vi "MH_SetHistoOnOff.vi"(8 "error in (no error)":errorcluster, 9 "tacq":i32, 10 "HistoOn/Off":bool, 11 "Multiharp in":refnum<class "Multiharp.lvclass">) -> (0 "error out":errorcluster, 3 "Multiharp out":refnum<class "Multiharp.lvclass">)   [LabVIEW 2023, in "SinglePhoton Library.lvlib" / "Multiharp.lvlib" / "Multiharp.lvclass"]
uses:
  Multiharp.lvclass
  Multiharp.lvclass/Multiharp.ctl
panel:
  in  "event data":T1
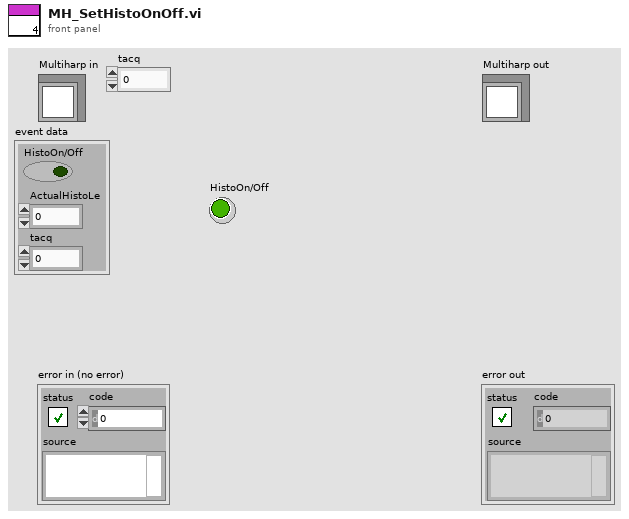
[diagram p1: front panel]
types:
  T1 = cluster{"HistoOn/Off":bool, "ActualHistoLe":i32, "tacq":i32}
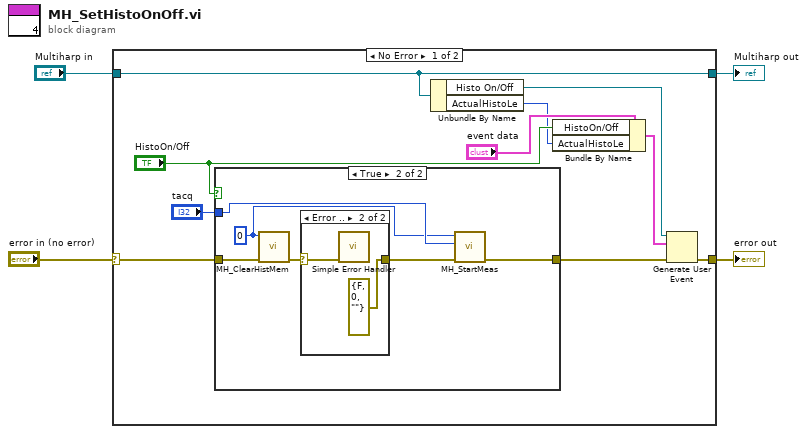
[diagram p0: block diagram]
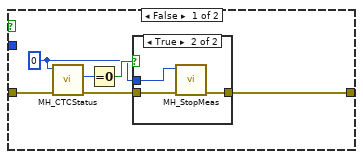
[diagram p2: hidden frame]
diagram:
  n1 = case shown="No Error" "error in (no error)" {
    selector: "error in (no error)" -> [w7 w35]
    tunnel: [w8 w35] -> w3
    tunnel: [w14 w34] -> w1
    tunnel: "Multiharp in" -> [w14 w34]
    frame No Error {
      n2 = case shown="True" "HistoOn/Off" {
        tunnel: [w18 w29] -> w9
        tunnel: w7 -> [w16 w28]
        tunnel: "tacq" -> [_ w30]
        frame False {
          w17 = 0 ("tacq")
          n3 = call "MH_CTCStatus.vi"("error in (no error)"=w16, "devidx"=w17) -> ("error out"=w15:errorcluster, "ctcstatus"=w20:i32)  [unwired: 7 in, 1 out]
          n4 = Equal To 0?(x=w20) -> (x = 0?=w19:bool)
          n5 = case shown="True" w19 {
            tunnel: w17 -> [_ w24]
            tunnel: w15 -> [w21 w23]
            tunnel: [w21 w22] -> w18
            frame False {
            }
            frame True {
              n6 = call "MH_StopMeas.vi"("error in (no error)"=w23, "devidx"=w24) -> ("error out"=w22:errorcluster)  [unwired: 8 in, 1 out]
            }
          }
        }
        frame True {
          w27 = 0 ("devidx")
          n7 = call "MH_ClearHistMem.vi"("error in (no error)"=w28, "devidx"=w27) -> ("error out"=w26:errorcluster)  [unwired: 8 in, 1 out]
          n8 = case shown="Error .." w26 {
            selector: w26 -> [w31 w32]
            tunnel: [w31 errorcluster {"status"=FALSE, "code"=0, "source"=""} ("error IO")] -> w25
            frame No Error {
            }
            frame Error {
              n9 = call <vilib>:"Simple Error Handler.vi"("error in (no error)"=w32) -> ()  [unwired: 4 in, 5 out]
            }
          }
          n10 = call "MH_StartMeas.vi"("error in (no error)"=w25, "tacq"=w30, "devidx"=w27) -> ("error out"=w29:errorcluster)  [unwired: 7 in, 1 out]
        }
      }
      n11 = Unbundle By Name(w14) -> ("Histo On/Off"=w6:refnum<user-event>, "ActualHistoLe"=w5:i32)
      n12 = Bundle By Name(cluster="event data", "HistoOn/Off"="HistoOn/Off", "ActualHistoLe"=w5) -> (w13:T1)
      n13 = Generate User Event(user event=w6, event data cluster=w13, error in=w9) -> (error out=w8:errorcluster)  [unwired: 1 in, 1 out]
    }
    frame Error {
    }
  }
  "error out" <- w3
  "Multiharp out" <- w1
